vi "oa_Perform Peak Averaging (1 Channel).vi"(6 "averaging state info out":T1 {"averages completed" format="%.2f"; "power spectrum" min=0.0 max=127.0 format="%.2f"; "complex FFT" format="%.2f"}, 7 "processing control in":T2(ring), 8 "error in (no error)":errorcluster, 9 "averaging parameters":T3={"averaging mode"=enum."No averaging", "weighting mode"=enum."Exponential", "number of averages"=10, "linear mode"=enum."One shot"} {"number of averages" min=1 step=1}, 11 "Y":dbl[][](array[numeric]) format="%.2f") -> (0 "error out":errorcluster, 1 "averages completed":dbl, 2 "averaging done":bool, 3 "Y out":dbl[](array[numeric]) format="%.2f", 4 "averaging state info out":T1 {"averages completed" format="%.2f"; "power spectrum" min=0.0 max=127.0 format="%.2f"; "complex FFT" format="%.2f"})   [LabVIEW 2017, in "SoundVib_Resampling.lvlib"]
uses:
  <vilib>/addons/Sound and Vibration/Order Analysis/Resample Order Tracking/SoundVib_Resampling.lvlib
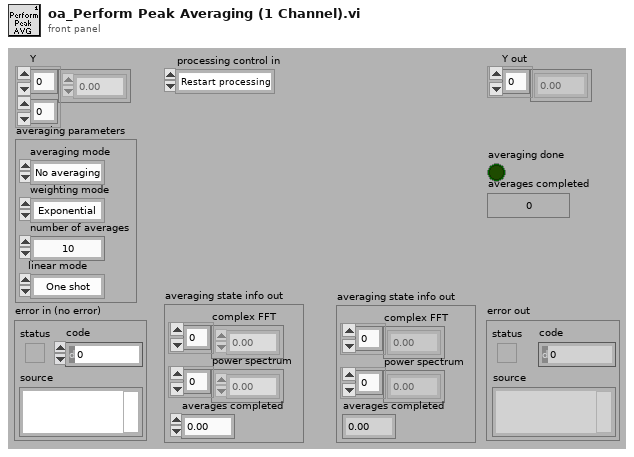
[diagram p1: front panel]
types:
  T1 = cluster{"complex FFT":cdb[], "power spectrum":dbl[], "averages completed":dbl}
  T2 = enum16{"Restart processing", "Continue processing", "Skip processing"}
  T3 = cluster{"averaging mode":enum16{"No averaging", "Vector averaging", "RMS averaging", "Peak hold"}, "weighting mode":enum16{"Linear", "Exponential"}, "number of averages":u32, "linear mode":enum16{"One shot", "Auto restart"}}
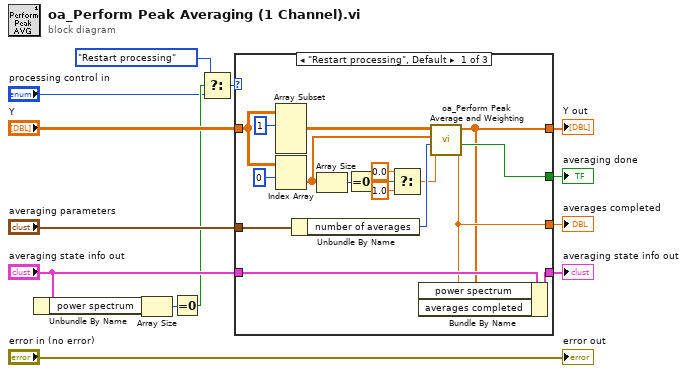
[diagram p0: block diagram]
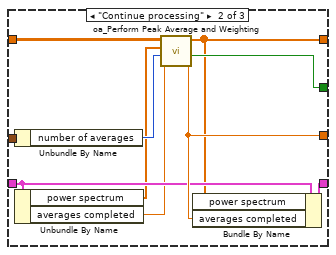
[diagram p2: hidden frame]
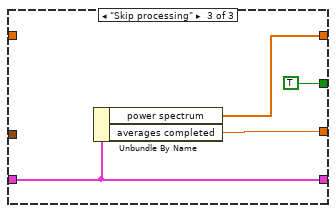
[diagram p3: hidden frame]
diagram:
  n1 = Unbundle By Name("averaging state info out") -> ("power spectrum"=w7:dbl[])
  n2 = Array Size(array=w7) -> (size(s)=w6:i32)
  n3 = Equal To 0?(x=w6) -> (x = 0?=w4:bool)
  n4 = Select(t=T2."Restart processing", s=w4, f="processing control in") -> (s? t:f=w1:T2)
  n5 = case shown="\"Restart processing\", Default" w1 {
    tunnel: "averaging parameters" -> [w29 w34 _]
    tunnel: "Y" -> [w18 w40 _]
    tunnel: "averaging state info out" -> [w31 w36 w44]
    tunnel: [w30 w37 w44] -> w12
    tunnel: [w26 w38 w43] -> w11
    tunnel: [w27 w39 TRUE] -> w10
    tunnel: [w25 w33 w42] -> w8
    frame "Restart processing", Default {
      n6 = Array Subset(array=w18, index (row)=1 ("index")) -> (w15:dbl[][])  [unwired: 3 in]
      n7 = Index Array(array=w18, index (row)=0) -> (element=w17:dbl[])  [unwired: 1 in]
      n8 = Unbundle By Name(w29) -> ("number of averages"=w28:u32)
      n9 = Array Size(array=w17) -> (size(s)=w22:i32)
      n10 = Equal To 0?(x=w22) -> (x = 0?=w19:bool)
      n11 = Select(t=0.0, s=w19, f=1.0) -> (s? t:f=w16:dbl)
      n12 = call <vilib>:"oa_Perform Peak Average and Weighting.vi"("averages completed"=w16, "number of averages"=w28, "previous array"=w17, "Y"=w15) -> ("averages completed out"=w26:dbl, "average done?"=w27:bool, "power spectrum"=w25:dbl[])  [unwired: 5 in]
      n13 = Bundle By Name(cluster=w31, "power spectrum"=w25, "averages completed"=w26) -> (w30:T1)
    }
    frame "Continue processing" {
      n14 = Unbundle By Name(w34) -> ("number of averages"=w41:u32)
      n15 = Unbundle By Name(w36) -> ("power spectrum"=w35:dbl[], "averages completed"=w32:dbl)
      n16 = call <vilib>:"oa_Perform Peak Average and Weighting.vi"("averages completed"=w32, "number of averages"=w41, "previous array"=w35, "Y"=w40) -> ("averages completed out"=w38:dbl, "average done?"=w39:bool, "power spectrum"=w33:dbl[])  [unwired: 5 in]
      n17 = Bundle By Name(cluster=w36, "power spectrum"=w33, "averages completed"=w38) -> (w37:T1)
    }
    frame "Skip processing" {
      n18 = Unbundle By Name(w44) -> ("power spectrum"=w42:dbl[], "averages completed"=w43:dbl)
    }
  }
  "averaging done" <- w10
  "averages completed" <- w11
  "Y out" <- w8
  "averaging state info out" <- w12
  "error out" <- "error in (no error)"
